vi "Forces.vi"() -> (1 "Fz":dbl, 2 "Fy":dbl, 3 "Fx":dbl)   [LabVIEW 2017]
uses:
  <userlib>/HapticSTM/Feedbackless - Testdata/HapticSTM.lvlib
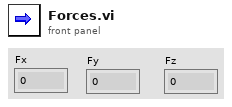
[diagram p1: front panel]
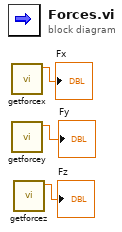
[diagram p0: block diagram]
diagram:
  n1 = call <userlib>:"getforcex.vi"() -> ("function return"=→"Fx":dbl)  [unwired: 11 in]
  n2 = call <userlib>:"getforcey.vi"() -> ("function return"=→"Fy":dbl)  [unwired: 11 in]
  n3 = call <userlib>:"getforcez.vi"() -> ("function return"=→"Fz":dbl)  [unwired: 11 in]
